vi "PathPlanner_PathFinder_GridPosToTranslation2d.vi"(11 "GridPosition":T1) -> (3 "RealGridPos":T2 {"Y" format="%14.3f"; "X" format="%14.3f"})   [LabVIEW 2019, in "PathPlanner24.lvlib"]
doc: "Internal function. Not to be used by end users."
uses:
  PathPlanner24.lvlib
  <vilib>/Rock Robotics/WPI/ThirdParty/JAS_Junk/TrajLib/TypeDef/TRANSLATION2D.ctl
  TypeDef/PathPlannerFinderGridPosition.ctl
  PathPlanner_PathFinder_Globals.vi
  <vilib>/Rock Robotics/WPI/ThirdParty/JAS_Junk/TrajLib/Trajectory_Library.lvlib
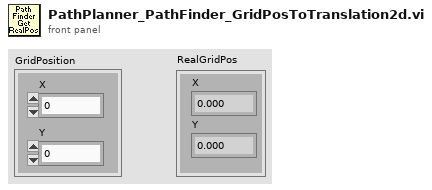
[diagram p1: front panel]
types:
  T1 = typedef "PathPlanner24.lvlib/PathPlannerFinderGridPosition.ctl" = cluster{"X":i32, "Y":i32}
  T2 = typedef "Trajectory_Library.lvlib/TRANSLATION2D.ctl" = cluster{"X":dbl, "Y":dbl}
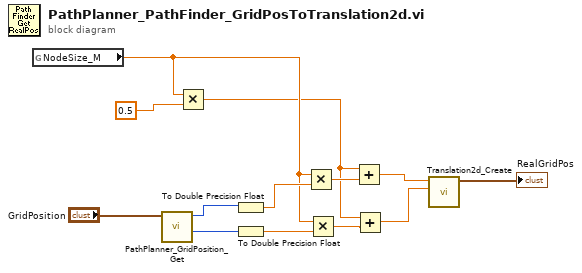
[diagram p0: block diagram]
diagram:
  n1 = global read "PathPlanner_PathFinder_Globals.vi" "NodeSize_M"() -> (w7:dbl)
  n2 = call "PathPlanner_GridPosition_Get.vi"("GridPosition"="GridPosition") -> ("Int Y"=w10:i32, "Int X"=w11:i32)  [unwired: 9 in]
  n3 = Multiply(x=w7, y=0.5 ("x")) -> (x*y=w4:dbl)
  n4 = To Double Precision Float(number=w11) -> (double precision float=w8:dbl)
  n5 = To Double Precision Float(number=w10) -> (double precision float=w9:dbl)
  n6 = Multiply(x=w7, y=w8) -> (x*y=w5:dbl)
  n7 = Multiply(x=w7, y=w9) -> (x*y=w6:dbl)
  n8 = Add(x=w4, y=w5) -> (x+y=w3:dbl)
  n9 = Add(x=w4, y=w6) -> (x+y=w2:dbl)
  n10 = call <vilib>:"Translation2d_Create.vi"("Y"=w2, "X"=w3) -> ("TRANSLATION"=→"RealGridPos":T2)  [unwired: 9 in]
